vi "Initialize Attributes.vi"(8 "error in (no error)":errorcluster, 10 "Attribute Data":variant, 11 "CS++GoBangServer in":refnum<class "CS++GoBangServer.lvclass">) -> (0 "error out":errorcluster, 2 "Found?":bool, 3 "CS++GoBangServer out":refnum<class "CS++GoBangServer.lvclass">)   [LabVIEW 2013, in "GoBang.lvlib" / "CS++GoBangServer.lvclass"]
doc: "Initialize object attribute.\n\nUnique resources should be allocated elsewhere!"
uses:
  CS++GoBangServer.lvclass
  Core/Classes/CS++ProcessVariables/SVConnection/SVConnection.lvclass
  Core/Actors/CS++BaseActor/CS++BaseActor.lvclass
  Core/Classes/CS++ProcessVariables/PVConnection/PVConnection.lvclass
  Core/Actors/CS++BaseActor/CS++BaseActor.lvclass/CS++BaseActor.ctl
  Core/Classes/CS++BaseClasses/Factory/CS++Factory.lvclass
  Core/Classes/CS++ProcessVariables/PVConnection/PVConnection.lvclass/PVConnection.ctl
  CS++GoBangServer.lvclass/CS++GoBangServer.ctl
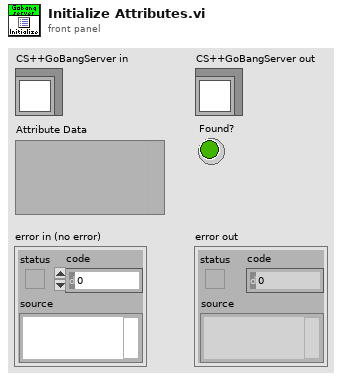
[diagram p1: front panel]
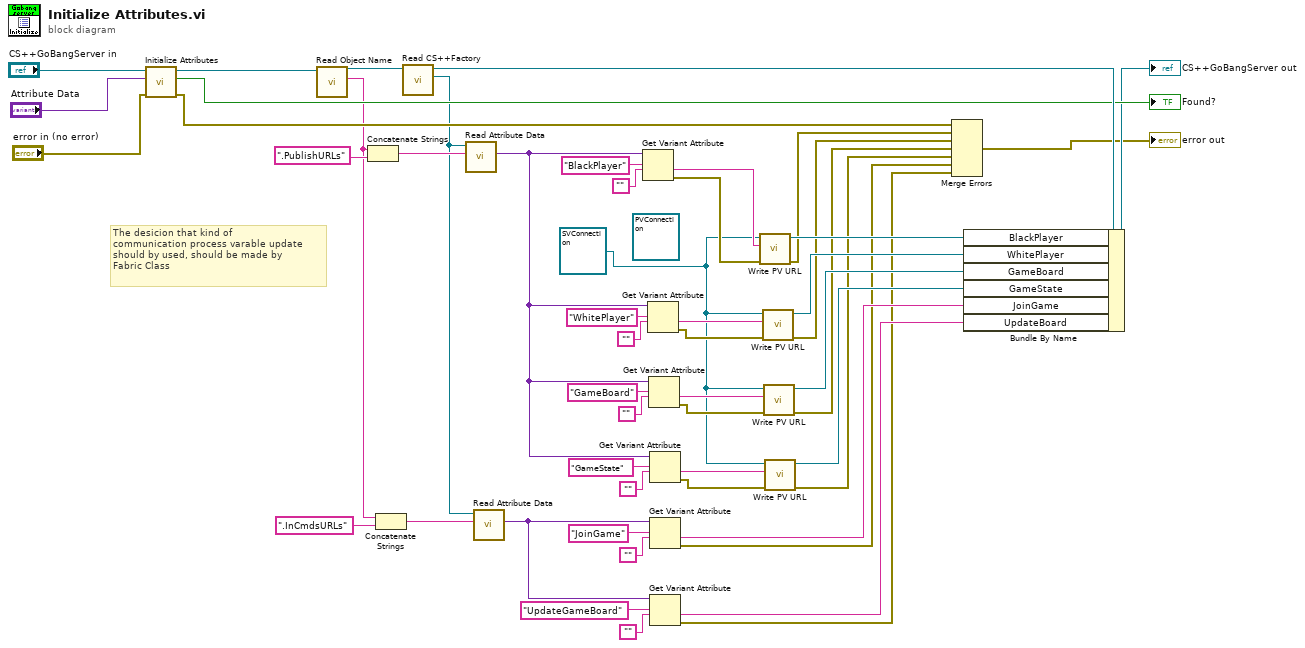
[diagram p0: block diagram]
diagram:
  w1 = refnum<class "SVConnection.lvclass"> refnum ("CS++ProcessVariables.lvlib:SVConnection.lvclass")
  (unwired) refnum<class "PVConnection.lvclass"> refnum ("CS++ProcessVariables.lvlib:PVConnection.lvclass")
  # "The desicion that kind of\ncommunication process varable update \nshould by used, should be made by \nFabric Class"
  n1 = call-parent "Initialize Attributes.vi"("error in (no error)"="error in (no error)", "Attribute Data"="Attribute Data", "CS++BaseActor in"="CS++GoBangServer in") -> ("error out"=w51:errorcluster, "Found?"=→"Found?":bool, "CS++BaseActor out"=w46:refnum<class "CS++GoBangServer.lvclass">)  [unwired: 6 in]
  n2 = call "Read Object Name.vi"("CS++BaseActor in"=w46) -> ("Object Name"=w13:string, "CS++BaseActor out"=w47:refnum<class "CS++GoBangServer.lvclass">)  [unwired: 8 in, 1 out]
  n3 = Concatenate Strings(w13, ".PublishURLs" ("string")) -> (w42:string)
  n4 = Concatenate Strings(w13, ".InCmdsURLs" ("string")) -> (w14:string)
  n5 = call "Read CS++Factory.vi"("CS++BaseActor in"=w47) -> ("CS++Factory"=w10:refnum<class "CS++Factory.lvclass">, "CS++BaseActor out"=w45:refnum<class "CS++GoBangServer.lvclass">)  [unwired: 8 in, 1 out]
  n6 = call-dynamic "Read Attribute Data.vi"("Object Name"=w42, "CS++Factory in"=w10) -> ("Attribute Data"=w20:variant)  [unwired: 7 in, 2 out]
  n7 = call-dynamic "Read Attribute Data.vi"("Object Name"=w14, "CS++Factory in"=w10) -> ("Attribute Data"=w5:variant)  [unwired: 7 in, 2 out]
  n8 = Get Variant Attribute(Variant=w20, name="BlackPlayer", default value (empty Variant)="") -> (value=w39:string, error out=w38:errorcluster)  [unwired: 1 in, 2 out]
  n9 = Get Variant Attribute(Variant=w20, name="WhitePlayer", default value (empty Variant)="") -> (value=w32:string, error out=w33:errorcluster)  [unwired: 1 in, 2 out]
  n10 = Get Variant Attribute(Variant=w20, name="GameBoard", default value (empty Variant)="") -> (value=w30:string, error out=w29:errorcluster)  [unwired: 1 in, 2 out]
  n11 = Get Variant Attribute(Variant=w20, name="GameState", default value (empty Variant)="") -> (value=w22:string, error out=w23:errorcluster)  [unwired: 1 in, 2 out]
  n12 = Get Variant Attribute(Variant=w5, name="JoinGame", default value (empty Variant)="") -> (value=w8:string, error out=w3:errorcluster)  [unwired: 1 in, 2 out]
  n13 = Get Variant Attribute(Variant=w5, name="UpdateGameBoard", default value (empty Variant)="") -> (value=w4:string, error out=w2:errorcluster)  [unwired: 1 in, 2 out]
  n14 = call "Write PV URL.vi"("error in (no error)"=w38, "PV URL"=w39, "PVConnection in"=w1) -> ("error out"=w18:errorcluster, "PVConnection out"=w36:refnum<class "SVConnection.lvclass">)  [unwired: 7 in]
  n15 = call "Write PV URL.vi"("error in (no error)"=w33, "PV URL"=w32, "PVConnection in"=w1) -> ("error out"=w17:errorcluster, "PVConnection out"=w31:refnum<class "SVConnection.lvclass">)  [unwired: 7 in]
  n16 = call "Write PV URL.vi"("error in (no error)"=w29, "PV URL"=w30, "PVConnection in"=w1) -> ("error out"=w16:errorcluster, "PVConnection out"=w26:refnum<class "SVConnection.lvclass">)  [unwired: 7 in]
  n17 = call "Write PV URL.vi"("error in (no error)"=w23, "PV URL"=w22, "PVConnection in"=w1) -> ("error out"=w15:errorcluster, "PVConnection out"=w21:refnum<class "SVConnection.lvclass">)  [unwired: 7 in]
  n18 = Merge Errors(w51, w18, w17, w16, w15, w3, w2) -> (→"error out":errorcluster)
  n19 = Bundle By Name(cluster=w45, "BlackPlayer"=w36, "WhitePlayer"=w31, "GameBoard"=w26, "GameState"=w21, "JoinGame"=w8, "UpdateBoard"=w4) -> (→"CS++GoBangServer out":refnum<class "CS++GoBangServer.lvclass">)
